vi "Initialize 3458A.vi"(7 "range [V] (10V)":dbl=10.0, 8 "error in (no error)":errorcluster, 10 "Reset (True)":bool, 11 "VISA DMM":refnum<visa-resource-name>) -> (0 "error out":errorcluster, 1 "sample memory [B]":i32, 2 "idn string":string, 3 "VISA resource name out":refnum<visa-resource-name>)   [LabVIEW 2013, in "3458A Virtual Digitizer.lvlib" / "3458A Digitizing Low Levels.lvlib"]
doc: "This VI does basic configuration of DMM for digitizing. It stops sampling, exports sync pulses to EXTOUT and does few more global settings that don't need to be changed for the measurement itself.\n\nNote: Reentrant VI so it can be executed in parallel for multiple 3458A sessions."
uses:
  3458A Digitizing Low Levels.lvlib
  3458A Basic Driver/3458A Basic Driver.lvlib
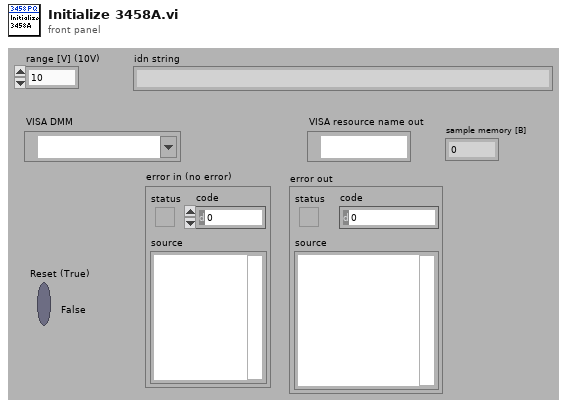
[diagram p1: front panel]
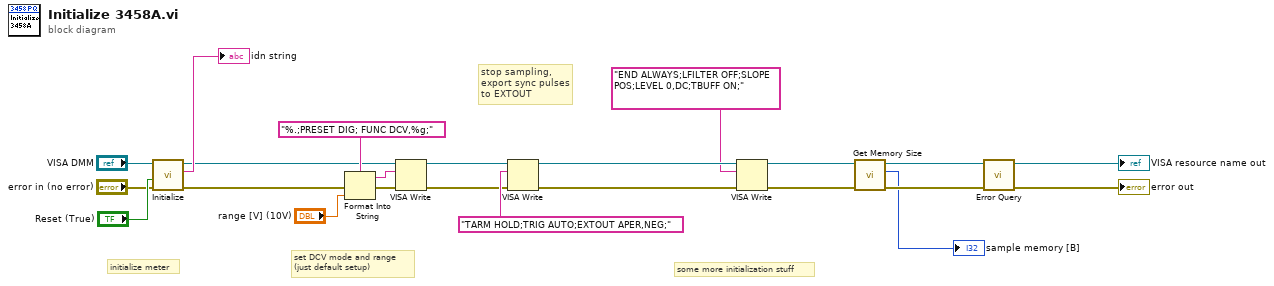
[diagram p0: block diagram]
diagram:
  # "some more initialization stuff"
  # "stop sampling,\nexport sync pulses\nto EXTOUT"
  # "set DCV mode and range\n(just default setup)"
  # "initialize meter"
  n1 = call "Initialize.vi"("error in (no error)"="error in (no error)", "Reset (True)"="Reset (True)", "VISA resource name"="VISA DMM") -> ("error out"=w12:errorcluster, "idn string"=→"idn string":string, "VISA resource name out"=w11:refnum<visa-resource-name>)  [unwired: 6 in]
  n2 = Format Into String(format string="%.;PRESET DIG; FUNC DCV,%g;" ("write buffer"), error in=w12, "range [V] (10V)") -> (resulting string=w18:string, error out=w19:errorcluster)  [unwired: 1 in]
  n3 = VISA Write(VISA resource name=w11, write buffer=w18, error in (no error)=w19) -> (VISA resource name out=w13:refnum<visa-resource-name>, error out=w14:errorcluster)  [unwired: 1 out]
  n4 = VISA Write(VISA resource name=w13, write buffer="TARM HOLD;TRIG AUTO;EXTOUT APER,NEG;", error in (no error)=w14) -> (VISA resource name out=w9:refnum<visa-resource-name>, error out=w10:errorcluster)  [unwired: 1 out]
  n5 = VISA Write(VISA resource name=w9, write buffer="END ALWAYS;LFILTER OFF;SLOPE POS;LEVEL 0,DC;TBUFF ON;", error in (no error)=w10) -> (VISA resource name out=w4:refnum<visa-resource-name>, error out=w5:errorcluster)  [unwired: 1 out]
  n6 = call "Get Memory Size.vi"("error in(no error)"=w5, "VISA Resource Name"=w4) -> ("error out"=w3:errorcluster, "sample memory [B]"=→"sample memory [B]":i32, "VISA resource name out"=w2:refnum<visa-resource-name>)  [unwired: 6 in, 1 out]
  n7 = call "Error Query.vi"("error in (no error)"=w3, "VISA resource name"=w2) -> ("error out"=→"error out":errorcluster, "VISA resource name out"=→"VISA resource name out":refnum<visa-resource-name>)  [unwired: 6 in, 2 out]
